vi "SeCrTs-RT_DAQ.vi"(8 "error in":errorcluster, 11 "Data FIFO Ref":T1) -> (0 "error out":errorcluster)   [LabVIEW 2022 SP3]
uses:
  RT Controls/SeCrTs-Data FIFO.ctl
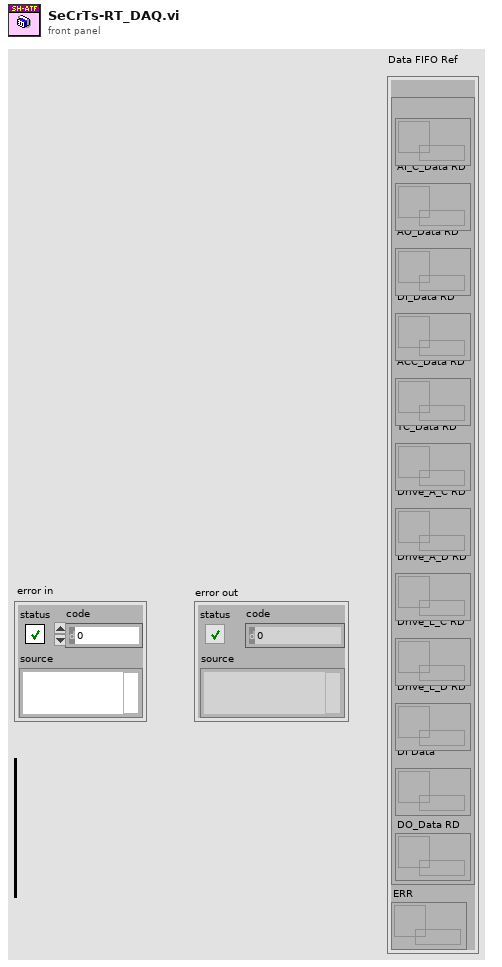
[diagram p1: front panel]
types:
  T1 = typedef "SeCrTs-Data FIFO.ctl" = cluster{"RD":cluster{"AI_V_Data RD":refnum<queue>, "AI_C_Data RD":refnum<queue>, "AO_Data RD":refnum<queue>, "DI_Data RD":refnum<queue>, "ACC_Data RD":refnum<queue>, "TC_Data RD":refnum<queue>, "Drive_A_C RD":refnum<queue>, "Drive_A_D RD":refnum<queue>, "Drive_L_C RD":refnum<queue>, "Drive_L_D RD":refnum<queue>, "DI Data":refnum<queue>, "DO_Data RD":refnum<queue>}, "ERR":refnum<queue>}
  T2 = cluster{"AO config":cluster{"Channel_Name":string, "Channel_Number":string, "Default_Value":dbl, "Units":string}[], "AI config":cluster{"Channel_Name":string, "Channel_Number":string, "Pre_Scale_min":dbl, "Pre_Scale_max":dbl, "Sensor_min":dbl, "Sensor_max":dbl, "Units":string}[], "DI config":cluster{"Channel_Name":string, "Channel_Number":string, "Default_Value":bool, "DI invert?":bool}[], "DO config":cluster{"Channel_Name":string, "Channel_Number":string, "Default_Value":bool, "DO invert?":bool}[], "TC config":cluster{"Channel_Name":string, "Channel_Number":string, "Pre_Scale_min":dbl, "Pre_Scale_max":dbl, "units":i32, " type":i32}[], "ACC config":cluster{"Channel_Name":string, "Channel_Number":string, "Pre_Scale_min":dbl, "Pre_Scale_max":dbl, "Terminal configuration":i32, "Sensitivity":dbl, "Sensitivity units":i32}[], "SG config":cluster{"Channel_Name":string, "Channel_Number":string, "Pre_Scale_min":dbl, "Pre_Scale_max":dbl}[], "Strain Gauge Settings":cluster{"poisson ratio":dbl, "nominal gage resistance":dbl, "gage factor":dbl}, "Bridge Settings":cluster{"voltage excitation value":dbl, "voltage excitation source":i32, "initial bridge voltage":dbl, "lead wire resistance":dbl, "strain configuration":i32}, "Sample Rate":cluster{"AI Sample Rate":dbl[], "AO Sample Rate":dbl[], "DI Sample Rate":dbl[], "TC Sample Rate":dbl[], "DO Sample Rate":dbl[], "SG Sample Rate":dbl[], "ACC Sample Rate":dbl[]}}
  T3 = enum16{"Initialize", "Create Task", "Start", "Acquire", "Stop", "Exit"}
  T4 = cluster{"AI_Task":refnum<k21>, "AO_Task":refnum<k21>, "DI_Task":refnum<k21>, "DO_Task":refnum<k21>, "ACC_Task":refnum<k21>, "TC_Task":refnum<k21>, "AI_V_Task":refnum<k21>}
  T5 = cluster{"Start DAQ":bool, "Stop DAQ":bool, "RT Stop":bool, "RT Exit":bool, "Start Seq":bool}
  T6 = cluster{"AO config":cluster{"Channel_Name":string, "Channel_Number":string, "Default_Value":dbl, "Units":string}[], "AI config":cluster{"Channel_Name":string, "Channel_Number":string, "Pre_Scale_min":dbl, "Pre_Scale_max":dbl, "Sensor_min":dbl, "Sensor_max":dbl, "Units":string}[], "DI config":cluster{"Channel_Name":string, "Channel_Number":string, "Default_Value":bool, "DI invert?":bool}[], "DO config":cluster{"Channel_Name":string, "Channel_Number":string, "Default_Value":bool, "DO invert?":bool}[], "TC config":cluster{"Channel_Name":string, "Channel_Number":string, "Pre_Scale_min":dbl, "Pre_Scale_max":dbl, "units":i32, "thermocouple type":i32}[], "ACC config":cluster{"Channel_Name":string, "Channel_Number":string, "Pre_Scale_min":dbl, "Pre_Scale_max":dbl, "Terminal configuration":i32, "Sensitivity":dbl, "Sensitivity units":i32}[], "SG config":cluster{"Channel_Name":string, "Channel_Number":string, "Pre_Scale_min":dbl, "Pre_Scale_max":dbl}[], "Strain Gauge Settings":cluster{"poisson ratio":dbl, "nominal gage resistance":dbl, "gage factor":dbl}, "Bridge Settings":cluster{"voltage excitation value":dbl, "voltage excitation source":i32, "initial bridge voltage":dbl, "lead wire resistance":dbl, "strain configuration":i32}, "Sample Rate":cluster{"AI Sample Rate":dbl[], "AO Sample Rate":dbl[], "DI Sample Rate":dbl[], "TC Sample Rate":dbl[], "DO Sample Rate":dbl[], "SG Sample Rate":dbl[], "ACC Sample Rate":dbl[]}}
  T7 = cluster{"Channel_Name":string, "Channel_Number":string, "Pre_Scale_min":dbl, "Pre_Scale_max":dbl, "Sensor_min":dbl, "Sensor_max":dbl, "Units":string}[]
  T8 = cluster{"Channel_Name":string, "Channel_Number":string, "Default_Value":dbl, "Units":string}[]
  T9 = cluster{"Channel_Name":string, "Channel_Number":string, "Default_Value":bool, "DI invert?":bool}[]
  T10 = cluster{"Channel_Name":string, "Channel_Number":string, "Default_Value":bool, "DO invert?":bool}[]
  T11 = cluster{"Channel_Name":string, "Channel_Number":string, "Pre_Scale_min":dbl, "Pre_Scale_max":dbl, "Terminal configuration":i32, "Sensitivity":dbl, "Sensitivity units":i32}[]
  T12 = cluster{"Channel_Name":string, "Channel_Number":string, "Pre_Scale_min":dbl, "Pre_Scale_max":dbl, "units":i32, " type":i32}[]
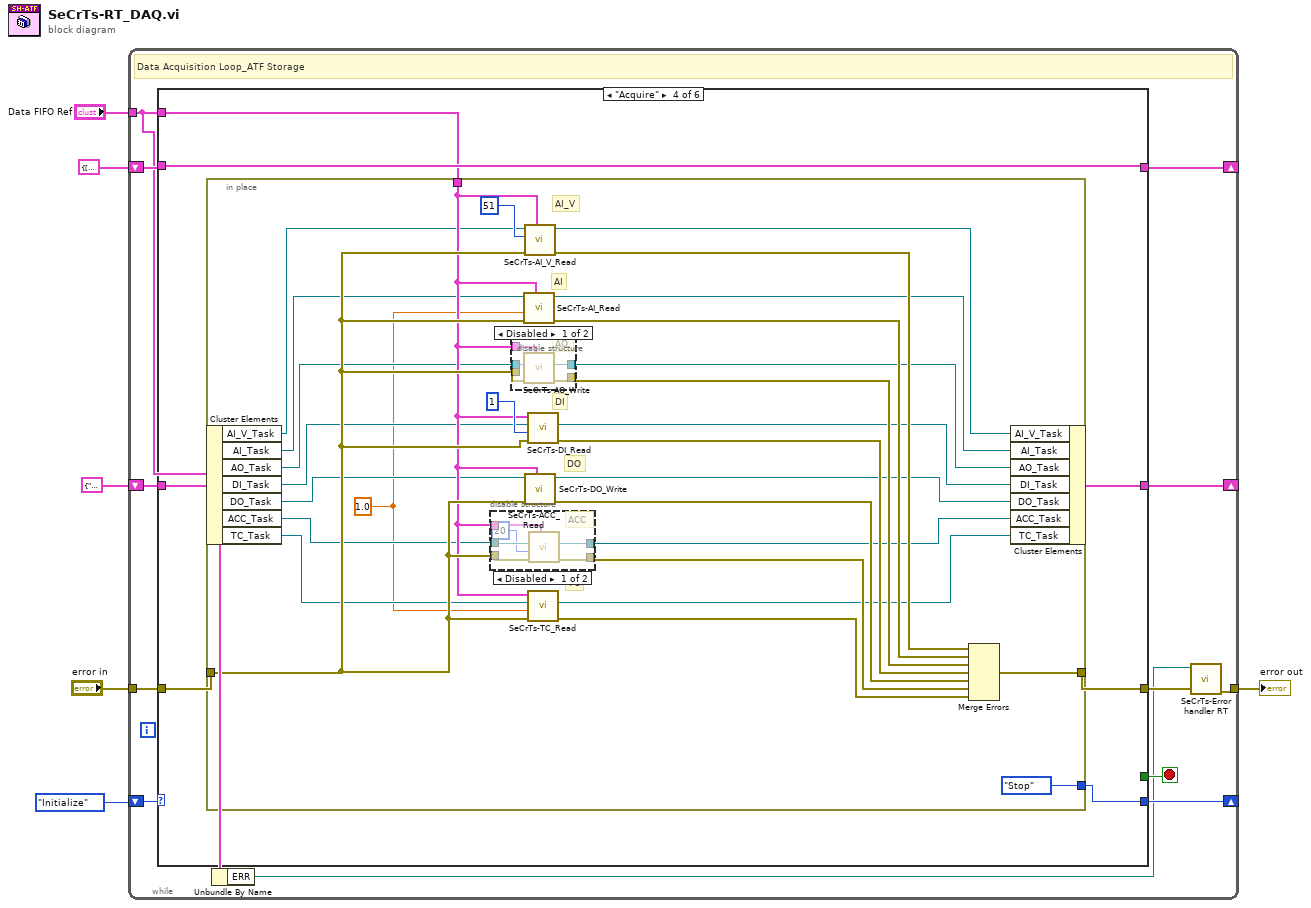
[diagram p0: block diagram]
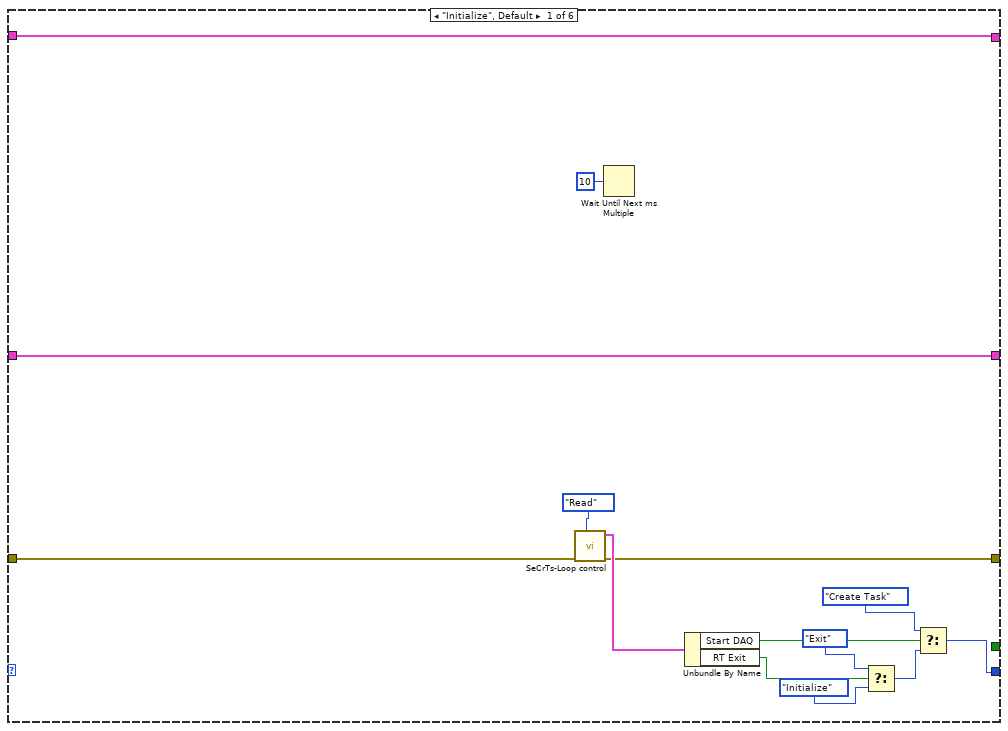
[diagram p2: hidden frame]
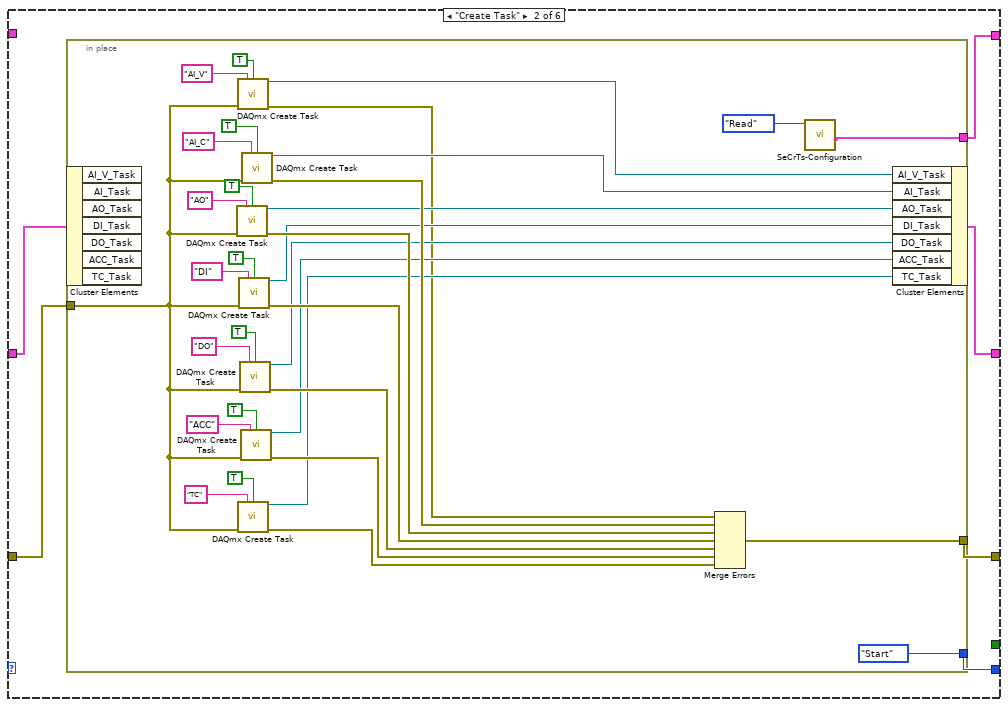
[diagram p3: hidden frame]
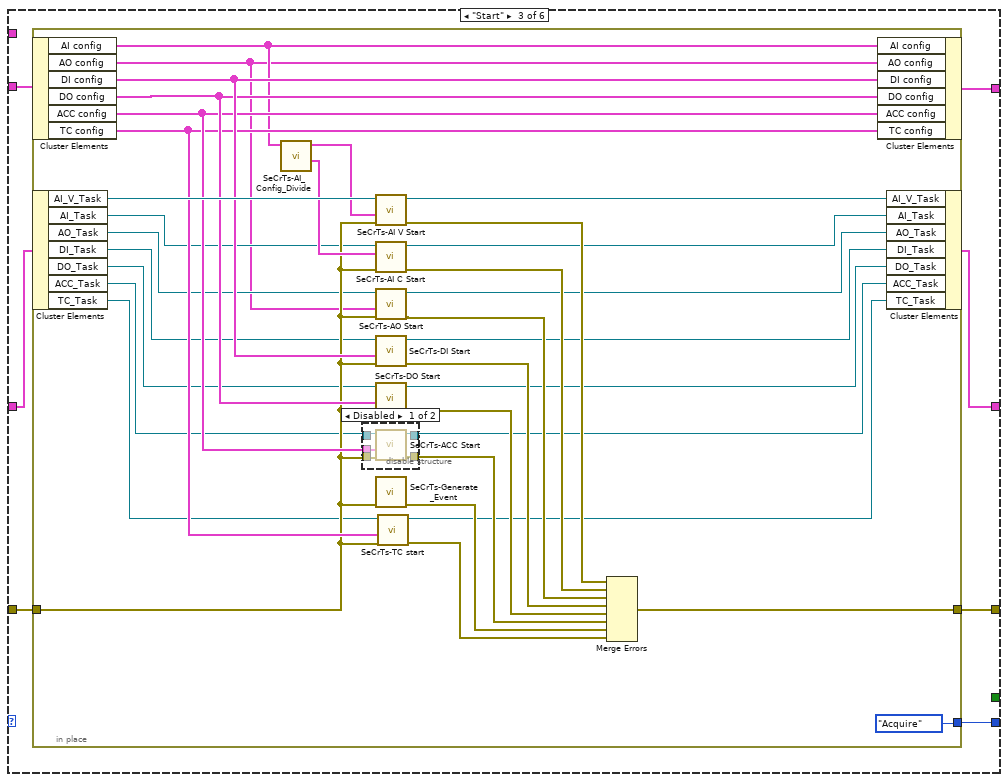
[diagram p4: hidden frame]
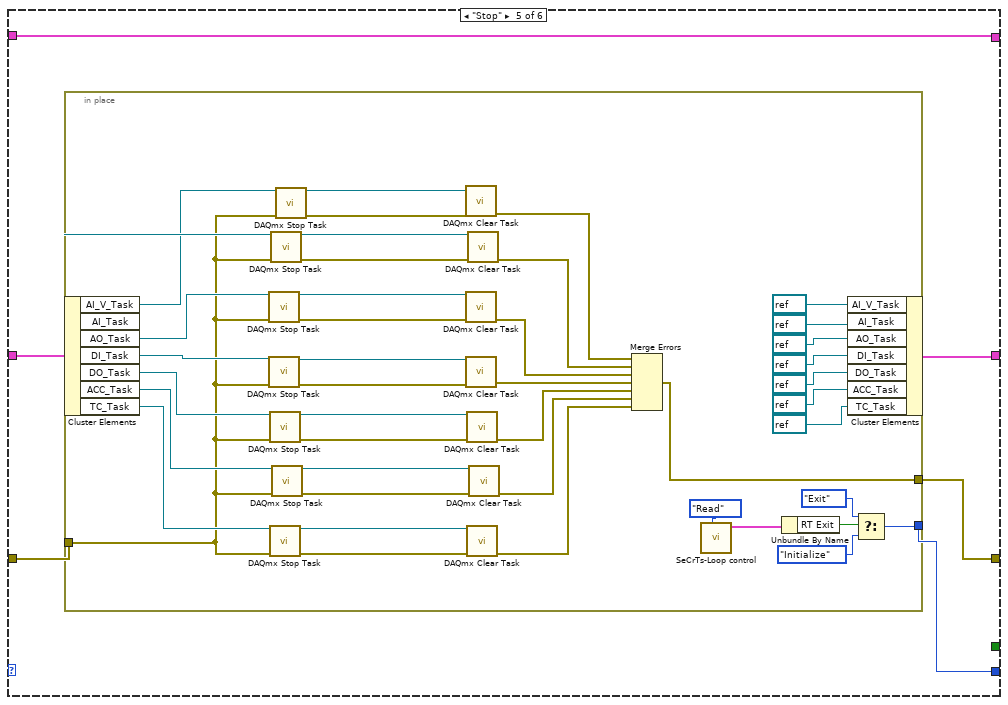
[diagram p8: hidden frame]
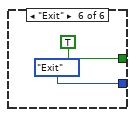
[diagram p9: hidden frame]
diagram:
  n1 = while {
    shift-right: [w16] -> _
    shift-left: T3."Initialize" -> [w18]
    tunnel: "error in" -> [w17]
    tunnel: [w9] -> w5
    shift-right: [w13] -> _
    shift-left: T2 {"AO config"=[], "AI config"=[], "DI config"=[], "DO config"=[], "TC config"=[], "ACC config"=[], "SG config"=[], "Strain Gauge Settings"={"poisson ratio"=0.0, "nominal gage resistance"=0.0, "gage factor"=0.0}, "Bridge Settings"={"voltage excitation value"=0.0, "voltage excitation source"=0, "initial bridge voltage"=0.0, "lead wire resistance"=0.0, "strain configuration"=0}, "Sample Rate"={"AI Sample Rate"=[], "AO Sample Rate"=[], "DI Sample Rate"=[], "TC Sample Rate"=[], "DO Sample Rate"=[], "SG Sample Rate"=[], "ACC Sample Rate"=[]}} ("Config out") -> [w14]
    shift-right: [w11] -> _
    shift-left: T4 {"AI_Task"="", "AO_Task"="", "DI_Task"="", "DO_Task"="", "ACC_Task"="", "TC_Task"="", "AI_V_Task"=""} -> [w15]
    tunnel: "Data FIFO Ref" -> [w8]
    stop <- w12 stop-if-true
    # "Data Acquisition Loop_ATF Storage"
    n2 = case shown="\"Acquire\"" w18 {
      tunnel: w17 -> [w21 w37 w77 w122 w166 _]
      tunnel: [w20 w36 w73 w121 w167 _] -> w10
      tunnel: [w31 w35 w78 w123 w168 T3."Exit"] -> w16
      tunnel: w15 -> [w23 w34 w76 w118 w165 _]
      tunnel: w14 -> [w22 _ w75 w120 w163 _]
      tunnel: [w22 w38 w74 w120 w163 _] -> w13
      tunnel: [_ _ _ _ _ TRUE] -> w12
      tunnel: [w23 w33 w72 w117 w164 _] -> w11
      tunnel: w8 -> [_ _ _ w119 _ _]
      frame "Initialize", Default {
        n3 = call "SeCrTs-Loop control.vi"("Action"=enum16{"Init", "Write", "Read"}."Read", "error in (no error)"=w21) -> ("error Out"=w20:errorcluster, "Loop Control out"=w27:T5)  [unwired: 8 in]
        n4 = Wait Until Next ms Multiple(millisecond multiple=u32 10) -> ()  [unwired: 1 out]
        n5 = Unbundle By Name(w27) -> ("Start DAQ"=w26:bool, "RT Exit"=w25:bool)
        n6 = Select(t=T3."Exit", s=w25, f=T3."Initialize") -> (s? t:f=w28:T3)
        n7 = Select(t=T3."Create Task", s=w26, f=w28) -> (s? t:f=w31:T3)
      }
      frame "Create Task" {
        n8 = in-place "In Place Element Structure" {
          in-place-border: [w50] -> w38
          in-place-border: w37 -> [w39]
          in-place-border: [w60] -> w36
          in-place-border: [T3."Start"] -> w35
          n9 = in-place-cluster #1(w34) -> ()  [unwired: 7 out]
          n10 = call <vilib>:"DAQmx Create Task.vi"("new task name"="AO", "auto cleanup"=TRUE, "error in"=w39) -> ("task out"=w58:refnum<k21>, "error out"=w65:errorcluster)  [unwired: 11 in]
          n11 = call <vilib>:"DAQmx Create Task.vi"("new task name"="AI_V", "auto cleanup"=TRUE, "error in"=w39) -> ("task out"=w51:refnum<k21>, "error out"=w40:errorcluster)  [unwired: 11 in]
          n12 = call <vilib>:"DAQmx Create Task.vi"("new task name"="TC", "auto cleanup"=TRUE, "error in"=w39) -> ("task out"=w54:refnum<k21>, "error out"=w61:errorcluster)  [unwired: 11 in]
          n13 = call <vilib>:"DAQmx Create Task.vi"("new task name"="DI", "auto cleanup"=TRUE, "error in"=w39) -> ("task out"=w57:refnum<k21>, "error out"=w64:errorcluster)  [unwired: 11 in]
          n14 = call <vilib>:"DAQmx Create Task.vi"("new task name"="DO", "auto cleanup"=TRUE, "error in"=w39) -> ("task out"=w56:refnum<k21>, "error out"=w63:errorcluster)  [unwired: 11 in]
          n15 = call <vilib>:"DAQmx Create Task.vi"("new task name"="ACC", "auto cleanup"=TRUE, "error in"=w39) -> ("task out"=w55:refnum<k21>, "error out"=w62:errorcluster)  [unwired: 11 in]
          n16 = call <vilib>:"DAQmx Create Task.vi"("new task name"="AI_C", "auto cleanup"=TRUE, "error in"=w39) -> ("task out"=w59:refnum<k21>, "error out"=w71:errorcluster)  [unwired: 11 in]
          n17 = Merge Errors(w40, w71, w65, w64, w63, w62, w61) -> (w60:errorcluster)
          n18 = call "SeCrTs-Configuration.vi"("Enum"=enum16{"Write", "Read"}."Read") -> ("Config out"=w50:T6)  [unwired: 10 in]
          n19 = in-place-cluster #1("AI_V_Task"=w51, "AI_Task"=w59, "AO_Task"=w58, "DI_Task"=w57, "DO_Task"=w56, "ACC_Task"=w55, "TC_Task"=w54) -> (w33:T4)
        }
      }
      frame "Start" {
        n20 = in-place "In Place Element Structure" {
          in-place-border: [T3."Acquire"] -> w78
          in-place-border: w77 -> [w97]
          in-place-border: [w92] -> w73
          n21 = in-place-cluster #2(w75) -> ("AI config"=w104:T7, "AO config"=w79:T8, "DI config"=w108:T9, "DO config"=w107:T10, "ACC config"=w106:T11, "TC config"=w105:T12)
          n22 = in-place-cluster #3(w76) -> ("AI_V_Task"=w110:refnum<k21>, "AI_Task"=w91:refnum<k21>, "AO_Task"=w90:refnum<k21>, "DI_Task"=w89:refnum<k21>, "DO_Task"=w88:refnum<k21>, "ACC_Task"=w87:refnum<k21>, "TC_Task"=w86:refnum<k21>)
          n23 = call "SeCrTs-AI_Config_Divide.vi"("AI config"=w104) -> ("AI C"=w102:T7, "AI V"=w103:T7)  [unwired: 9 in]
          n24 = disable-structure shown="Disabled" {
            disable-tunnel: w106 -> [w116 _]
            disable-tunnel: w97 -> [w115 _]
            disable-tunnel: [w114 _] -> w95
            disable-tunnel: w87 -> [w113 _]
            disable-tunnel: [w112 _] -> w81
            frame Disabled {
              n25 = call "SeCrTs-ACC Start.vi"("error in"=w115, "ACC config"=w116, "Refnum in"=w113) -> ("error out"=w114:errorcluster, "Refnum out"=w112:refnum<k21>)  [unwired: 7 in]
            }
            frame Enabled {
            }
          }
          n26 = call "SeCrTs-AI V Start .vi"("error in"=w97, "AI V"=w103, "Refnum in"=w110) -> ("error out"=w101:errorcluster, "Refnum out"=w109:refnum<k21>)  [unwired: 7 in]
          n27 = call "SeCrTs-AI C Start .vi"("error in"=w97, "AI C"=w102, "Refnum in"=w91) -> ("error out"=w100:errorcluster, "Refnum out"=w85:refnum<k21>)  [unwired: 7 in]
          n28 = call "SeCrTs-AO Start .vi"("error in"=w97, "AO config"=w79, "Refnum in"=w90) -> ("error out"=w99:errorcluster, "Refnum out"=w84:refnum<k21>)  [unwired: 7 in]
          n29 = call "SeCrTs-DI Start.vi"("error in"=w97, "DI config"=w108, "Refnum in"=w89) -> ("error out"=w98:errorcluster, "Refnum out"=w83:refnum<k21>)  [unwired: 7 in]
          n30 = call "SeCrTs-DO Start.vi"("error in"=w97, "DO config"=w107, "Refnum in"=w88) -> ("error out"=w96:errorcluster, "Refnum out"=w82:refnum<k21>)  [unwired: 7 in]
          n31 = call "SeCrTs-Generate_Event.vi"("error in"=w97) -> ("error out"=w94:errorcluster)  [unwired: 10 in]
          n32 = call "SeCrTs-TC start .vi"("error in"=w97, "TC config"=w105, "Refnum in"=w86) -> ("error out"=w93:errorcluster, "Refnum out"=w80:refnum<k21>)  [unwired: 7 in]
          n33 = Merge Errors(w101, w100, w99, w98, w96, w95, w94, w93) -> (w92:errorcluster)
          n34 = in-place-cluster #2("AI config"=w104, "AO config"=w79, "DI config"=w108, "DO config"=w107, "ACC config"=w106, "TC config"=w105) -> (w74:T2)
          n35 = in-place-cluster #3("AI_V_Task"=w109, "AI_Task"=w85, "AO_Task"=w84, "DI_Task"=w83, "DO_Task"=w82, "ACC_Task"=w81, "TC_Task"=w80) -> (w72:T4)
        }
      }
      frame "Acquire" {
        n36 = in-place "In Place Element Structure" {
          in-place-border: [T3."Stop"] -> w123
          in-place-border: w122 -> [w142]
          in-place-border: [w150] -> w121
          in-place-border: w119 -> [w140]
          w124 = 1.0
          # "AI_V"
          # "TC"
          # "DO"
          # "DI"
          # "AI"
          n37 = in-place-cluster #4(w118) -> ("AI_V_Task"=w125:refnum<k21>, "AI_Task"=w139:refnum<k21>, "AO_Task"=w138:refnum<k21>, "DI_Task"=w137:refnum<k21>, "DO_Task"=w136:refnum<k21>, "ACC_Task"=w135:refnum<k21>, "TC_Task"=w134:refnum<k21>)
          n38 = disable-structure shown="Disabled" {
            disable-tunnel: [w157 _] -> w144
            disable-tunnel: w142 -> [w156 _]
            disable-tunnel: w140 -> [w155 _]
            disable-tunnel: w135 -> [w154 _]
            disable-tunnel: [w153 _] -> w128
            frame Disabled {
              # "ACC"
              n39 = call "SeCrTs-ACC_Read.vi"("Data FIFO Ref"=w155, "error in (no error)"=w156, "number of samples per channel"=20, "ACC_Task"=w154) -> ("error out"=w157:errorcluster, "task out"=w153:refnum<k21>)  [unwired: 6 in]
            }
            frame Enabled {
            }
          }
          n40 = disable-structure shown="Disabled" {
            disable-tunnel: [w162 _] -> w147
            disable-tunnel: w142 -> [w161 _]
            disable-tunnel: w140 -> [w160 _]
            disable-tunnel: w138 -> [w159 _]
            disable-tunnel: [w158 _] -> w131
            frame Disabled {
              # "AO"
              n41 = call "SeCrTs-AO_Write.vi"("Data FIFO Ref"=w160, "error in (no error)"=w161, "AO_Task"=w159) -> ("error out"=w162:errorcluster, "task out"=w158:refnum<k21>)  [unwired: 7 in]
            }
            frame Enabled {
            }
          }
          n42 = call "SeCrTs-AI_Read.vi"("Data FIFO Ref"=w140, "error in (no error)"=w142, "Numeric"=w124, "AI_Task"=w139) -> ("error out"=w148:errorcluster, "task out"=w132:refnum<k21>)  [unwired: 4 in]
          n43 = call "SeCrTs-AI_V_Read.vi"("Data FIFO Ref"=w140, "error in"=w142, "number of samples per channel"=51, "AI_V_Task"=w125) -> ("error out"=w149:errorcluster, "AI_V_Task"=w133:refnum<k21>)  [unwired: 6 in]
          n44 = call "SeCrTs-DO_Write.vi"("Data FIFO Ref"=w140, "error in (no error)"=w142, "Refnum in"=w136) -> ("error out"=w145:errorcluster, "Refnum out"=w129:refnum<k21>)  [unwired: 7 in]
          n45 = call "SeCrTs-DI_Read.vi"("error in (no error)"=w142, "number of samples per channel"=1, "DI_Task"=w137, "Data FIFO Ref"=w140) -> ("error out"=w146:errorcluster, "task out"=w130:refnum<k21>)  [unwired: 6 in]
          n46 = call "SeCrTs-TC_Read.vi"("error in (no error)"=w142, "Numeric"=w124, "TC_Task"=w134, "Data FIFO Ref"=w140) -> ("error out"=w143:errorcluster, "task out"=w127:refnum<k21>)  [unwired: 6 in]
          n47 = Merge Errors(w149, w148, w147, w146, w145, w144, w143) -> (w150:errorcluster)
          n48 = in-place-cluster #4("AI_V_Task"=w133, "AI_Task"=w132, "AO_Task"=w131, "DI_Task"=w130, "DO_Task"=w129, "ACC_Task"=w128, "TC_Task"=w127) -> (w117:T4)
        }
      }
      frame "Stop" {
        n49 = in-place "In Place Element Structure" {
          in-place-border: [w208] -> w168
          in-place-border: [w202] -> w167
          in-place-border: w166 -> [w183]
          n50 = in-place-cluster #5(w165) -> ("AI_V_Task"=w185:refnum<k21>, "AI_Task"=w194:refnum<k21>, "AO_Task"=w193:refnum<k21>, "DI_Task"=w196:refnum<k21>, "DO_Task"=w195:refnum<k21>, "ACC_Task"=w192:refnum<k21>, "TC_Task"=w191:refnum<k21>)
          n51 = call <vilib>:"DAQmx Stop Task.vi"("task/channels in"=w193, "error in"=w183) -> ("task out"=w190:refnum<k21>, "error out"=w207:errorcluster)  [unwired: 12 in]
          n52 = call <vilib>:"DAQmx Stop Task.vi"("task/channels in"=w196, "error in"=w183) -> ("task out"=w189:refnum<k21>, "error out"=w206:errorcluster)  [unwired: 12 in]
          n53 = call <vilib>:"DAQmx Stop Task.vi"("task/channels in"=w195, "error in"=w183) -> ("task out"=w188:refnum<k21>, "error out"=w205:errorcluster)  [unwired: 12 in]
          n54 = call <vilib>:"DAQmx Stop Task.vi"("task/channels in"=w191, "error in"=w183) -> ("task out"=w186:refnum<k21>, "error out"=w203:errorcluster)  [unwired: 12 in]
          n55 = call <vilib>:"DAQmx Stop Task.vi"("task/channels in"=w194, "error in"=w183) -> ("task out"=w171:refnum<k21>, "error out"=w170:errorcluster)  [unwired: 12 in]
          n56 = call <vilib>:"DAQmx Stop Task.vi"("task/channels in"=w192, "error in"=w183) -> ("task out"=w187:refnum<k21>, "error out"=w204:errorcluster)  [unwired: 12 in]
          n57 = call <vilib>:"DAQmx Stop Task.vi"("task/channels in"=w185, "error in"=w183) -> ("task out"=w184:refnum<k21>, "error out"=w182:errorcluster)  [unwired: 12 in]
          n58 = call <vilib>:"DAQmx Clear Task.vi"("task in"=w184, "error in"=w182) -> ("error out"=w181:errorcluster)  [unwired: 13 in]
          n59 = call <vilib>:"DAQmx Clear Task.vi"("task in"=w190, "error in"=w207) -> ("error out"=w201:errorcluster)  [unwired: 13 in]
          n60 = call <vilib>:"DAQmx Clear Task.vi"("task in"=w189, "error in"=w206) -> ("error out"=w200:errorcluster)  [unwired: 13 in]
          n61 = call <vilib>:"DAQmx Clear Task.vi"("task in"=w188, "error in"=w205) -> ("error out"=w199:errorcluster)  [unwired: 13 in]
          n62 = call <vilib>:"DAQmx Clear Task.vi"("task in"=w186, "error in"=w203) -> ("error out"=w197:errorcluster)  [unwired: 13 in]
          n63 = call <vilib>:"DAQmx Clear Task.vi"("task in"=w171, "error in"=w170) -> ("error out"=w211:errorcluster)  [unwired: 13 in]
          n64 = call <vilib>:"DAQmx Clear Task.vi"("task in"=w187, "error in"=w204) -> ("error out"=w198:errorcluster)  [unwired: 13 in]
          n65 = Merge Errors(w181, w211, w201, w200, w199, w198, w197) -> (w202:errorcluster)
          n66 = call "SeCrTs-Loop control.vi"("Action"=enum16{"Init", "Write", "Read"}."Read") -> ("Loop Control out"=w180:T5)  [unwired: 9 in, 1 out]
          n67 = Unbundle By Name(w180) -> ("RT Exit"=w179:bool)
          n68 = in-place-cluster #5("AI_V_Task"=refnum<k21> refnum, "AI_Task"=refnum<k21> refnum, "AO_Task"=refnum<k21> refnum, "DI_Task"=refnum<k21> refnum, "DO_Task"=refnum<k21> refnum, "ACC_Task"=refnum<k21> refnum, "TC_Task"=refnum<k21> refnum) -> (w164:T4)
          n69 = Select(t=T3."Exit", s=w179, f=T3."Initialize") -> (s? t:f=w208:T3)
        }
      }
      frame "Exit" {
      }
    }
    n70 = Unbundle By Name(w8) -> ("ERR"=w7:refnum<queue>)
    n71 = call "SeCrTs-Error handler RT.vi"("error in"=w10, "Message Queue"=w7) -> ("error out"=w9:errorcluster)  [unwired: 8 in, 1 out]
  }
  "error out" <- w5
